vi "Apply.vi"(8 "error in":errorcluster, 11 "PXI-5441 Base CFG in":refnum<class "DC CFG.lvclass">) -> (0 "error out":errorcluster, 3 "PXI-5441 Base CFG out":refnum<class "DC CFG.lvclass">)   [LabVIEW 2023, in "PXI-5441.lvlib" / "DC CFG.lvclass"]
uses:
  DC CFG.lvclass
  DC CFG.lvclass/DC CFG.ctl
  Fgen PXI/Fgen PXI CFG/Fgen PXI CFG.lvclass
  D:/git/HAL/Fgen PXI/Fgen PXI CFG/Fgen PXI CFG.lvclass
  D:/git/HAL/Configuration Base/Configuration Base.lvclass
  D:/git/HAL/Interfaces/IConfigure/IConfigure.lvclass
  D:/git/HAL/Devices/PXI-5441/Configurations/DC CFG/DC CFG.lvclass
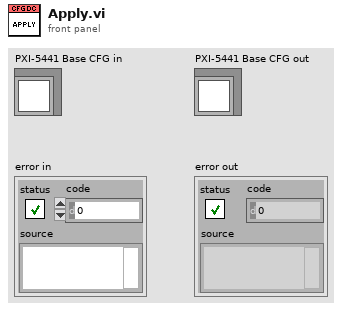
[diagram p1: front panel]
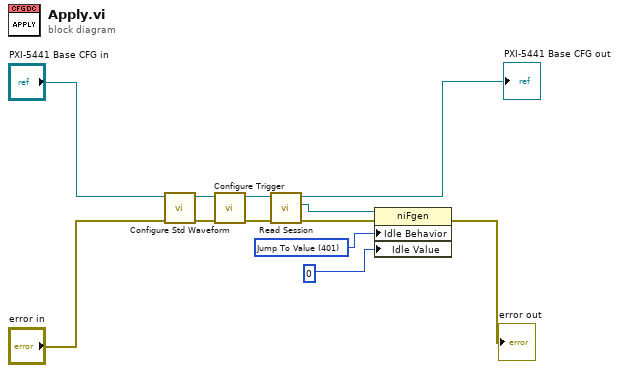
[diagram p0: block diagram]
diagram:
  w2 = 401 items=["Hold Last Value"=400, "Jump To Value"=401] ("Output:Advanced:Idle Behavior")
  n1 = call-dynamic "Configure Std Waveform.vi"("error in"="error in", "PXI-5441 Base CFG in"="PXI-5441 Base CFG in") -> ("error out"=w9:errorcluster, "PXI-5441 Base CFG out"=w10:refnum<class "DC CFG.lvclass">)  [unwired: 8 in]
  n2 = call "Configure Trigger.vi"("error in"=w9, "PXI-5441 Base CFG in"=w10) -> ("error out"=w8:errorcluster, "PXI-5441 Base CFG out"=w6:refnum<class "DC CFG.lvclass">)  [unwired: 8 in]
  n3 = call "Read Session.vi"("error in (no error)"=w8, "Fgen PXI CFG in"=w6) -> ("error out"=w7:errorcluster, "Session"=w3:refnum<k15>, "Fgen PXI CFG out"=→"PXI-5441 Base CFG out":refnum<class "DC CFG.lvclass">)  [unwired: 7 in]
  n4 = property class="niFgen"(reference=w3, error in=w7, "Idle Behavior"=w2, "Idle Value"=0 ("Output:Advanced:Idle Value")) -> (error out=→"error out":errorcluster)  [unwired: 1 out]
